vi "储运信息检索.vi"(3 "大于/小于":bool, 4 "检索数据":ext=2.0, 5 "检索项":enum16{"ID", "Tmperature"}(ring)=enum."Tmperature", 6 "connection reference":T2) -> (0 "error out":errorcluster caption="错误输出", 1 "检索信息":T1(array[cluster]), 2 "布尔":bool)   [LabVIEW 2018]
uses:
  <vilib>/addons/database/Connection.llb/Conn ObjectReference.ctl
  <vilib>/addons/database/_DB Variant To Data/Database Variant To Data.xnode
  <vilib>/addons/database/NI_Database_API.lvlib
panel:
  in  "停止":bool
  # "检索储运信息"
  # "大于"
  # "小于"
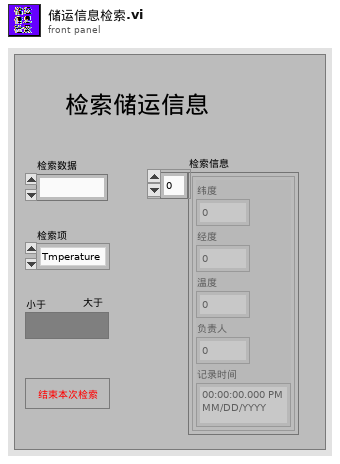
[diagram p1: front panel]
types:
  T1 = cluster{"纬度":sgl, "经度":sgl, "温度":sgl, "负责人":i32, "记录时间":timestamp}[]
  T2 = typedef "NI_Database_API.lvlib/Conn ObjectReference.ctl" = refnum<k1>
  T3 = typedef "储运信息.ctl" = cluster{"纬度":sgl, "经度":sgl, "温度":sgl, "负责人":i32, "区域":string, "记录时间":timestamp}
  T4 = enum8{"Enabled", "Disabled", "Disabled and Grayed Out"}
  T5 = cluster{"纬度":sgl, "经度":sgl, "温度":sgl, "负责人":i32, "记录时间":timestamp}
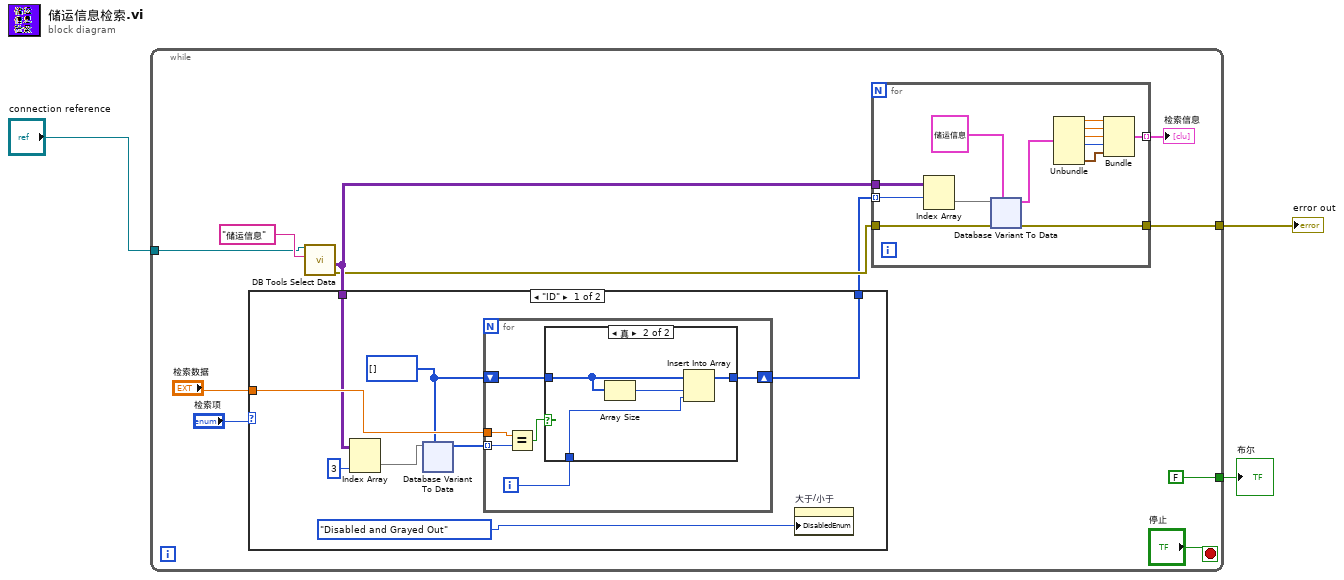
[diagram p0: block diagram]
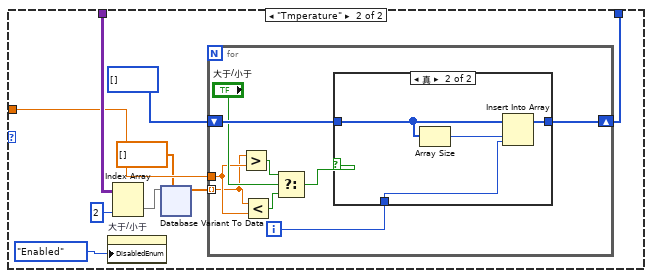
[diagram p3: hidden frame]
diagram:
  n1 = while {
    tunnel: [w10] -> w3
    tunnel: "connection reference" -> [w7]
    tunnel: [FALSE] -> w1
    stop <- "停止" stop-if-true
    n2 = call <vilib>:"DB Tools Select Data.vi"("table"="储运信息", "connection reference"=w7) -> ("error out"=w11:errorcluster, "data"=w12:variant[][])  [unwired: 4 in, 1 out]
    n3 = case shown="\"ID\"" "检索项" {
      tunnel: "检索数据" -> [w236 w290]
      tunnel: w12 -> [w235 w292]
      tunnel: [w232 w291] -> w8
      frame "ID" {
        w233 = i32[] []
        n4 = Index Array(array=w235, index (col)=3 ("禁用的索引 (列)")) -> (element=w238:variant[])  [unwired: 1 in]
        n5 = xnode "Database Variant To Data"("database variant"=w238, "type"=w233) -> ("data"=w237:i32[])  [unwired: 1 in, 1 out]
        n6 = for {
          tunnel: w237 -> [w243] mode=indexing
          tunnel: w236 -> [w244]
          shift-right: [w239] -> w232
          shift-left: w233 -> [w240]
          i -> [w241]
          n7 = Equal?(x=w244, y=w243) -> (x = y?=w242:bool)
          n8 = case shown="真" w242 {
            tunnel: w241 -> [_ w248]
            tunnel: w240 -> [w245 w247]
            tunnel: [w245 w249] -> w239
            frame False {
            }
            frame True {
              n9 = Array Size(array=w247) -> (size(s)=w246:i32)
              n10 = Insert Into Array(array=w247, index=w246, new element=w248) -> (w249:i32[])
            }
          }
        }
        n11 = property on="大于/小于" class="Bool (严格)"("DisabledEnum"=T4."Disabled and Grayed Out" ("禁用")) -> ()  [unwired: 2 in, 2 out]
      }
      frame "Tmperature" {
        n12 = property on="大于/小于" class="Bool (严格)"("DisabledEnum"=T4."Enabled" ("禁用")) -> ()  [unwired: 2 in, 2 out]
        n13 = Index Array(array=w292, index (col)=2 ("禁用的索引 (列)")) -> (element=w296:variant[])  [unwired: 1 in]
        n14 = xnode "Database Variant To Data"("database variant"=w296, "type"=dbl[] []) -> ("data"=w295:dbl[])  [unwired: 1 in, 1 out]
        n15 = for {
          tunnel: w295 -> [w297] mode=indexing
          tunnel: w290 -> [w298]
          shift-right: [w303] -> w291
          shift-left: i32[] [] -> [w304]
          i -> [w305]
          n16 = Greater?(x=w297, y=w298) -> (0:w301:bool)
          n17 = Less?(x=w297, y=w298) -> (x < y?=w300:bool)
          n18 = Select(t=w301, s="大于/小于", f=w300) -> (s? t:f=w299:bool)
          n19 = case shown="真" w299 {
            tunnel: w305 -> [_ w310]
            tunnel: w304 -> [w306 w308]
            tunnel: [w306 w309] -> w303
            frame False {
            }
            frame True {
              n20 = Array Size(array=w308) -> (size(s)=w307:i32)
              n21 = Insert Into Array(array=w308, index=w307, new element=w310) -> (w309:i32[])
            }
          }
        }
      }
    }
    n22 = for {
      tunnel: w12 -> [w25]
      tunnel: w8 -> [w22] mode=indexing
      tunnel: w11 -> [w24]
      tunnel: [w23] -> w10
      tunnel: [w15] -> w6 mode=indexing
      n23 = Index Array(array=w25, index (row)=w22) -> (element=w27:variant[])  [unwired: 1 in]
      n24 = xnode "Database Variant To Data"("database variant"=w27, "error in (no error)"=w24, "type"=T3 {"纬度"=0.0, "经度"=0.0, "温度"=0.0, "负责人"=0, "区域"="", "记录时间"=timestamp(0 s since 1904-01-01)} ("簇")) -> ("data"=w21:T3, "error out"=w23:errorcluster)
      n25 = Unbundle(w21) -> ("纬度"=w20:sgl, "经度"=w19:sgl, "温度"=w18:sgl, "负责人"=w17:i32, "记录时间"=w16:timestamp)  [unwired: 1 out]
      n26 = Bundle("纬度"=w20, "经度"=w19, "温度"=w18, "负责人"=w17, "记录时间"=w16) -> (w15:T5)  [unwired: 1 in]
    }
    "检索信息" <- w6
  }
  "error out" <- w3
  "布尔" <- w1
